vi "SequenceSelector_LoadAllChambers.vi"(5 "Inflow Channel Selector":dbl, 9 "Loop Iteration":i32) -> (4 "Array":u8[][](array[numeric])=[[0, 0, 0, 0, 0, 0, 0, 0, 2, 4, 3, 3, 3, 3], [0, 0, 0, 0, 0, 0, 0, 0, 0, 0, 0, 0, 0, 0], [0, 0, 0, 0, 0, 0, 0, 0, 0, 0, 0, 0, 0, 0], [0, 0, 0, 0, 0, 0, 0, 0, 0, 0, 0, 0, 0, 0], [0, 0, 0, 0, 0, 0, 0, 0, 0, 0, 0, 0, 0, 0], [11, 11, 11, 11, 11, 11, 11, 0, 0, 0, 0, 0, 0, 0], [0, 0, 0, 0, 0, 0, 0, 0, 0, 0, 0, 0, 0, 0], [16, 16, 16, 16, 16, 16, 16, 0, 0, 0, 0, 0, 0, 0], [0, 0, 0, 0, 0, 0, 0, 0, 0, 0, 0, 0, 0, 0], [0, 0, 0, 0, 0, 0, 0, 0, 0, 0, 0, 0, 0, 0], [0, 0, 0, 0, 0, 0, 0, 0, 0, 0, 0, 0, 0, 0], [2, 2, 2, 2, 2, 2, 2, 0, 0, 0, 0, 0, 0, 0], [4, 4, 4, 4, 4, 4, 4, 0, 0, 0, 0, 0, 0, 0], [255, 255, 255, 255, 255, 255, 0, 0, 0, 0, 0, 0, 0, 0], [3, 2, 6, 4, 5, 1, 0, 0, 0, 0, 0, 0, 0, 0], [31, 31, 31, 31, 31, 31, 0, 0, 0, 0, 0, 0, 0, 0], [255, 255, 255, 255, 255, 255, 0, 0, 0, 0, 0, 0, 0, 0]])   [LabVIEW 2016]
panel:
  in  "Byte 4":dbl[](array[numeric])
  in  "Byte 3":dbl[](array[numeric])
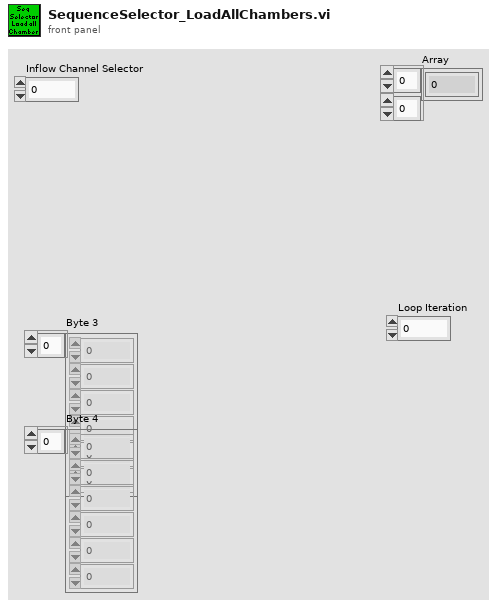
[diagram p1: front panel]
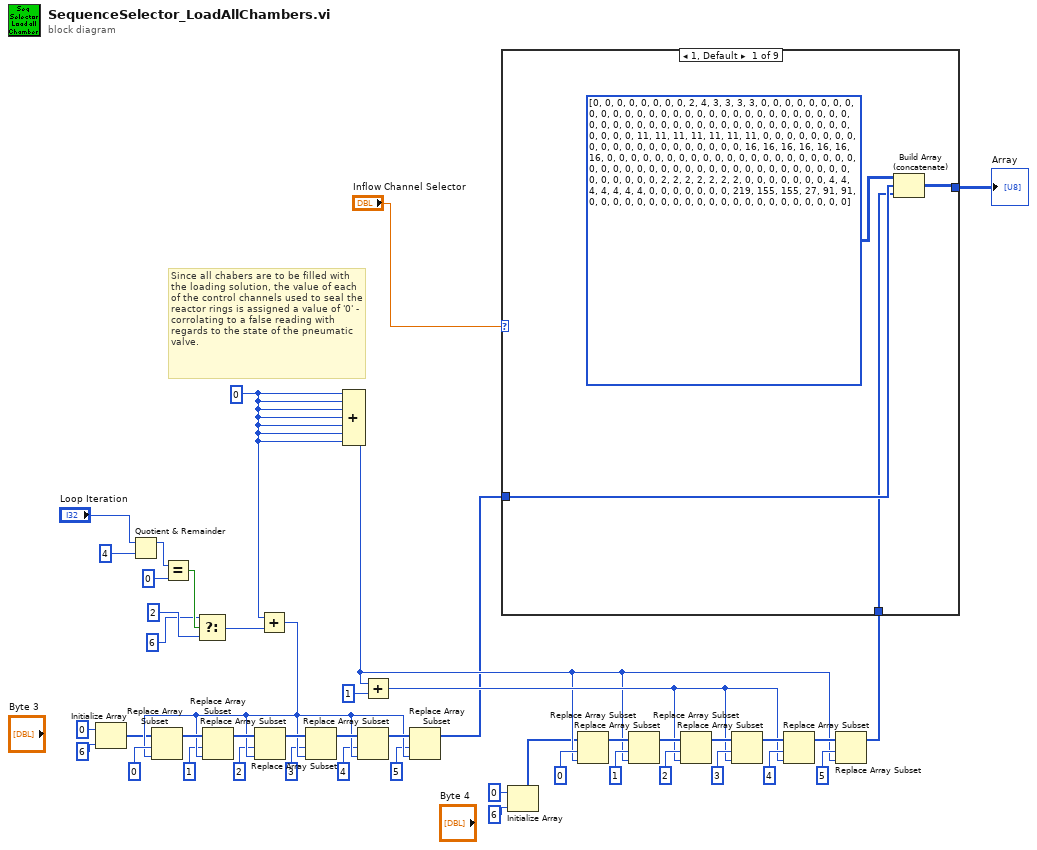
[diagram p0: block diagram]
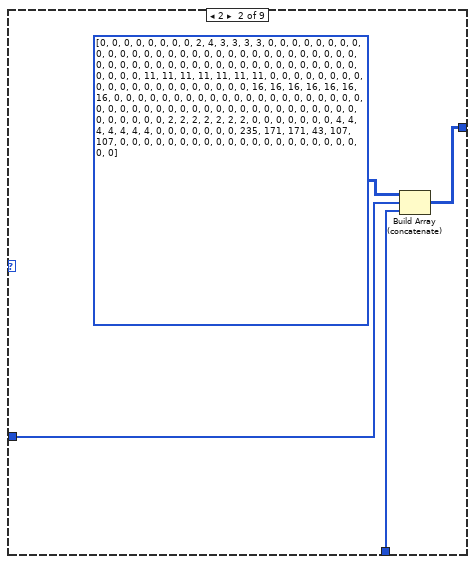
[diagram p2: hidden frame]
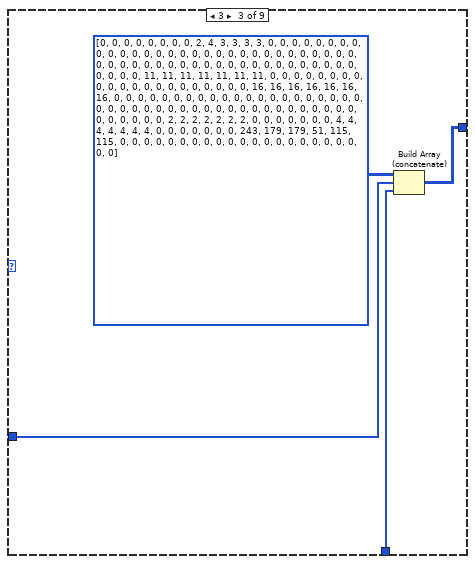
[diagram p3: hidden frame]
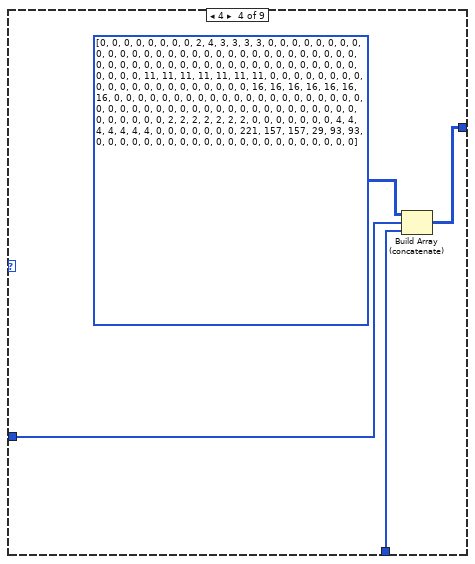
[diagram p4: hidden frame]
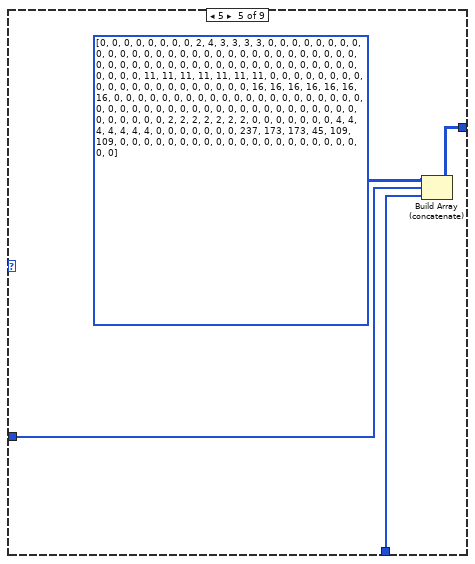
[diagram p5: hidden frame]
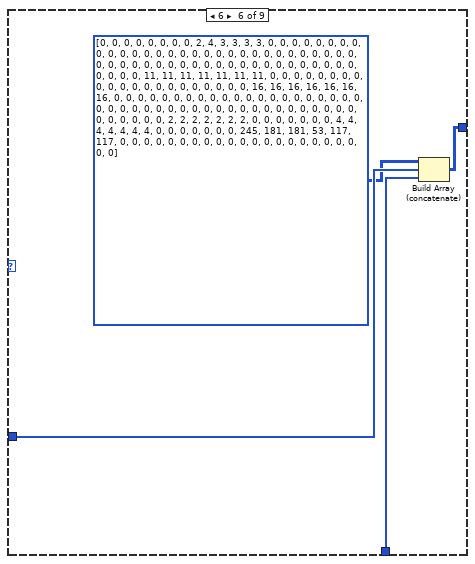
[diagram p6: hidden frame]
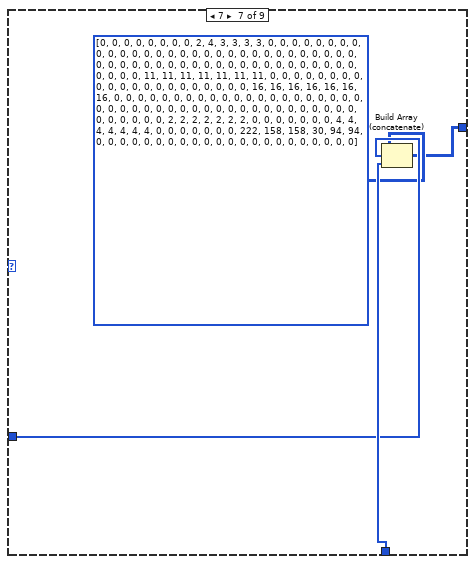
[diagram p7: hidden frame]
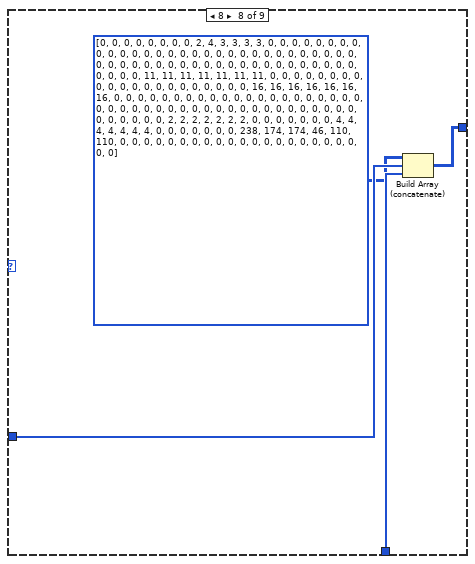
[diagram p8: hidden frame]
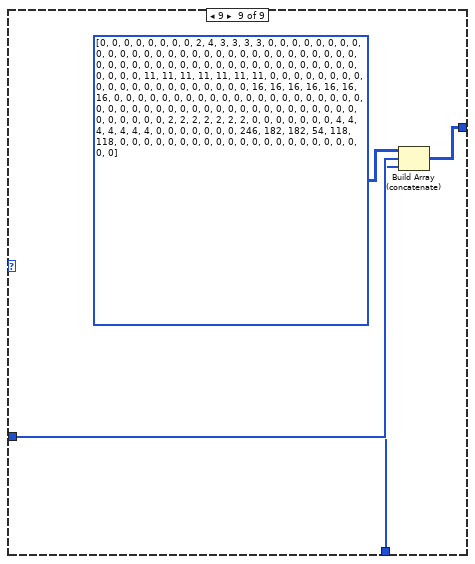
[diagram p9: hidden frame]
diagram:
  w9 = 0
  # "Since all chabers are to be filled with the loading solution, the value of each of the control channels used to seal the reactor rings is assigned a value of '0' - corrolating to a false reading with regards to the state of the pneumatic valve."
  n1 = Initialize Array(0, 6) -> (w10:i32[])
  n2 = Quotient & Remainder(x="Loop Iteration", y=4) -> (x-y*floor(x/y)=w1:i32)  [unwired: 1 out]
  n3 = Equal?(x=w1, y=0) -> (x = y?=w8:bool)
  n4 = Select(t=6, s=w8, f=2) -> (s? t:f=w3:i32)
  n5 = Add(x=w9, y=w3) -> (x+y=w38:i32)
  n6 = Replace Array Subset(array=w10, new element=w38, index=0) -> (w43:i32[])
  n7 = Replace Array Subset(array=w43, new element=w38, index=1) -> (w42:i32[])
  n8 = Replace Array Subset(array=w42, new element=w38, index=2) -> (w41:i32[])
  n9 = Replace Array Subset(array=w41, new element=w38, index=3) -> (w40:i32[])
  n10 = Compound Arithmetic op=unknown(w9, w9, w9, w9, w9, w9, w9) -> (w19:i32)
  n11 = Replace Array Subset(array=w40, new element=w38, index=4) -> (w39:i32[])
  n12 = Add(x=w19, y=1) -> (x+y=w20:i32)
  n13 = Replace Array Subset(array=w39, new element=w38, index=5) -> (w18:i32[])
  n14 = Initialize Array(0, 6) -> (w15:i32[])
  n15 = Replace Array Subset(array=w15, new element=w19, index=0) -> (w23:i32[])
  n16 = Replace Array Subset(array=w23, new element=w19, index=1) -> (w24:i32[])
  n17 = Replace Array Subset(array=w24, new element=w20, index=2) -> (w25:i32[])
  n18 = Replace Array Subset(array=w25, new element=w20, index=3) -> (w26:i32[])
  n19 = Replace Array Subset(array=w26, new element=w20, index=4) -> (w27:i32[])
  n20 = Replace Array Subset(array=w27, new element=w19, index=5) -> (w17:i32[])
  n21 = case shown="1, Default" "Inflow Channel Selector" {
    tunnel: [w49 w50 w54 w58 w65 w69 w70 w74 w80] -> w16
    tunnel: w18 -> [w47 w52 w56 w60 w63 w67 w72 w76 w79]
    tunnel: w17 -> [w46 w53 w57 w61 w64 w68 w73 w77 w78]
    frame 1, Default {
      n22 = Build Array (concatenate)(u8[][] [[0, 0, 0, 0, 0, 0, 0, 0, 2, 4, 3, 3, 3, 3], [0, 0, 0, 0, 0, 0, 0, 0, 0, 0, 0, 0, 0, 0], [0, 0, 0, 0, 0, 0, 0, 0, 0, 0, 0, 0, 0, 0], [0, 0, 0, 0, 0, 0, 0, 0, 0, 0, 0, 0, 0, 0], [0, 0, 0, 0, 0, 0, 0, 0, 0, 0, 0, 0, 0, 0], [11, 11, 11, 11, 11, 11, 11, 0, 0, 0, 0, 0, 0, 0], [0, 0, 0, 0, 0, 0, 0, 0, 0, 0, 0, 0, 0, 0], [16, 16, 16, 16, 16, 16, 16, 0, 0, 0, 0, 0, 0, 0], [0, 0, 0, 0, 0, 0, 0, 0, 0, 0, 0, 0, 0, 0], [0, 0, 0, 0, 0, 0, 0, 0, 0, 0, 0, 0, 0, 0], [0, 0, 0, 0, 0, 0, 0, 0, 0, 0, 0, 0, 0, 0], [2, 2, 2, 2, 2, 2, 2, 0, 0, 0, 0, 0, 0, 0], [4, 4, 4, 4, 4, 4, 4, 0, 0, 0, 0, 0, 0, 0], [219, 155, 155, 27, 91, 91, 0, 0, 0, 0, 0, 0, 0, 0], [0, 0, 0, 0, 0, 0, 0, 0, 0, 0, 0, 0, 0, 0]], w47, w46) -> (w49:i32[][])
    }
    frame 2 {
      n23 = Build Array (concatenate)(u8[][] [[0, 0, 0, 0, 0, 0, 0, 0, 2, 4, 3, 3, 3, 3], [0, 0, 0, 0, 0, 0, 0, 0, 0, 0, 0, 0, 0, 0], [0, 0, 0, 0, 0, 0, 0, 0, 0, 0, 0, 0, 0, 0], [0, 0, 0, 0, 0, 0, 0, 0, 0, 0, 0, 0, 0, 0], [0, 0, 0, 0, 0, 0, 0, 0, 0, 0, 0, 0, 0, 0], [11, 11, 11, 11, 11, 11, 11, 0, 0, 0, 0, 0, 0, 0], [0, 0, 0, 0, 0, 0, 0, 0, 0, 0, 0, 0, 0, 0], [16, 16, 16, 16, 16, 16, 16, 0, 0, 0, 0, 0, 0, 0], [0, 0, 0, 0, 0, 0, 0, 0, 0, 0, 0, 0, 0, 0], [0, 0, 0, 0, 0, 0, 0, 0, 0, 0, 0, 0, 0, 0], [0, 0, 0, 0, 0, 0, 0, 0, 0, 0, 0, 0, 0, 0], [2, 2, 2, 2, 2, 2, 2, 0, 0, 0, 0, 0, 0, 0], [4, 4, 4, 4, 4, 4, 4, 0, 0, 0, 0, 0, 0, 0], [235, 171, 171, 43, 107, 107, 0, 0, 0, 0, 0, 0, 0, 0], [0, 0, 0, 0, 0, 0, 0, 0, 0, 0, 0, 0, 0, 0]], w52, w53) -> (w50:i32[][])
    }
    frame 3 {
      n24 = Build Array (concatenate)(u8[][] [[0, 0, 0, 0, 0, 0, 0, 0, 2, 4, 3, 3, 3, 3], [0, 0, 0, 0, 0, 0, 0, 0, 0, 0, 0, 0, 0, 0], [0, 0, 0, 0, 0, 0, 0, 0, 0, 0, 0, 0, 0, 0], [0, 0, 0, 0, 0, 0, 0, 0, 0, 0, 0, 0, 0, 0], [0, 0, 0, 0, 0, 0, 0, 0, 0, 0, 0, 0, 0, 0], [11, 11, 11, 11, 11, 11, 11, 0, 0, 0, 0, 0, 0, 0], [0, 0, 0, 0, 0, 0, 0, 0, 0, 0, 0, 0, 0, 0], [16, 16, 16, 16, 16, 16, 16, 0, 0, 0, 0, 0, 0, 0], [0, 0, 0, 0, 0, 0, 0, 0, 0, 0, 0, 0, 0, 0], [0, 0, 0, 0, 0, 0, 0, 0, 0, 0, 0, 0, 0, 0], [0, 0, 0, 0, 0, 0, 0, 0, 0, 0, 0, 0, 0, 0], [2, 2, 2, 2, 2, 2, 2, 0, 0, 0, 0, 0, 0, 0], [4, 4, 4, 4, 4, 4, 4, 0, 0, 0, 0, 0, 0, 0], [243, 179, 179, 51, 115, 115, 0, 0, 0, 0, 0, 0, 0, 0], [0, 0, 0, 0, 0, 0, 0, 0, 0, 0, 0, 0, 0, 0]], w56, w57) -> (w54:i32[][])
    }
    frame 4 {
      n25 = Build Array (concatenate)(u8[][] [[0, 0, 0, 0, 0, 0, 0, 0, 2, 4, 3, 3, 3, 3], [0, 0, 0, 0, 0, 0, 0, 0, 0, 0, 0, 0, 0, 0], [0, 0, 0, 0, 0, 0, 0, 0, 0, 0, 0, 0, 0, 0], [0, 0, 0, 0, 0, 0, 0, 0, 0, 0, 0, 0, 0, 0], [0, 0, 0, 0, 0, 0, 0, 0, 0, 0, 0, 0, 0, 0], [11, 11, 11, 11, 11, 11, 11, 0, 0, 0, 0, 0, 0, 0], [0, 0, 0, 0, 0, 0, 0, 0, 0, 0, 0, 0, 0, 0], [16, 16, 16, 16, 16, 16, 16, 0, 0, 0, 0, 0, 0, 0], [0, 0, 0, 0, 0, 0, 0, 0, 0, 0, 0, 0, 0, 0], [0, 0, 0, 0, 0, 0, 0, 0, 0, 0, 0, 0, 0, 0], [0, 0, 0, 0, 0, 0, 0, 0, 0, 0, 0, 0, 0, 0], [2, 2, 2, 2, 2, 2, 2, 0, 0, 0, 0, 0, 0, 0], [4, 4, 4, 4, 4, 4, 4, 0, 0, 0, 0, 0, 0, 0], [221, 157, 157, 29, 93, 93, 0, 0, 0, 0, 0, 0, 0, 0], [0, 0, 0, 0, 0, 0, 0, 0, 0, 0, 0, 0, 0, 0]], w60, w61) -> (w58:i32[][])
    }
    frame 5 {
      n26 = Build Array (concatenate)(u8[][] [[0, 0, 0, 0, 0, 0, 0, 0, 2, 4, 3, 3, 3, 3], [0, 0, 0, 0, 0, 0, 0, 0, 0, 0, 0, 0, 0, 0], [0, 0, 0, 0, 0, 0, 0, 0, 0, 0, 0, 0, 0, 0], [0, 0, 0, 0, 0, 0, 0, 0, 0, 0, 0, 0, 0, 0], [0, 0, 0, 0, 0, 0, 0, 0, 0, 0, 0, 0, 0, 0], [11, 11, 11, 11, 11, 11, 11, 0, 0, 0, 0, 0, 0, 0], [0, 0, 0, 0, 0, 0, 0, 0, 0, 0, 0, 0, 0, 0], [16, 16, 16, 16, 16, 16, 16, 0, 0, 0, 0, 0, 0, 0], [0, 0, 0, 0, 0, 0, 0, 0, 0, 0, 0, 0, 0, 0], [0, 0, 0, 0, 0, 0, 0, 0, 0, 0, 0, 0, 0, 0], [0, 0, 0, 0, 0, 0, 0, 0, 0, 0, 0, 0, 0, 0], [2, 2, 2, 2, 2, 2, 2, 0, 0, 0, 0, 0, 0, 0], [4, 4, 4, 4, 4, 4, 4, 0, 0, 0, 0, 0, 0, 0], [237, 173, 173, 45, 109, 109, 0, 0, 0, 0, 0, 0, 0, 0], [0, 0, 0, 0, 0, 0, 0, 0, 0, 0, 0, 0, 0, 0]], w63, w64) -> (w65:i32[][])
    }
    frame 6 {
      n27 = Build Array (concatenate)(u8[][] [[0, 0, 0, 0, 0, 0, 0, 0, 2, 4, 3, 3, 3, 3], [0, 0, 0, 0, 0, 0, 0, 0, 0, 0, 0, 0, 0, 0], [0, 0, 0, 0, 0, 0, 0, 0, 0, 0, 0, 0, 0, 0], [0, 0, 0, 0, 0, 0, 0, 0, 0, 0, 0, 0, 0, 0], [0, 0, 0, 0, 0, 0, 0, 0, 0, 0, 0, 0, 0, 0], [11, 11, 11, 11, 11, 11, 11, 0, 0, 0, 0, 0, 0, 0], [0, 0, 0, 0, 0, 0, 0, 0, 0, 0, 0, 0, 0, 0], [16, 16, 16, 16, 16, 16, 16, 0, 0, 0, 0, 0, 0, 0], [0, 0, 0, 0, 0, 0, 0, 0, 0, 0, 0, 0, 0, 0], [0, 0, 0, 0, 0, 0, 0, 0, 0, 0, 0, 0, 0, 0], [0, 0, 0, 0, 0, 0, 0, 0, 0, 0, 0, 0, 0, 0], [2, 2, 2, 2, 2, 2, 2, 0, 0, 0, 0, 0, 0, 0], [4, 4, 4, 4, 4, 4, 4, 0, 0, 0, 0, 0, 0, 0], [245, 181, 181, 53, 117, 117, 0, 0, 0, 0, 0, 0, 0, 0], [0, 0, 0, 0, 0, 0, 0, 0, 0, 0, 0, 0, 0, 0]], w67, w68) -> (w69:i32[][])
    }
    frame 7 {
      n28 = Build Array (concatenate)(u8[][] [[0, 0, 0, 0, 0, 0, 0, 0, 2, 4, 3, 3, 3, 3], [0, 0, 0, 0, 0, 0, 0, 0, 0, 0, 0, 0, 0, 0], [0, 0, 0, 0, 0, 0, 0, 0, 0, 0, 0, 0, 0, 0], [0, 0, 0, 0, 0, 0, 0, 0, 0, 0, 0, 0, 0, 0], [0, 0, 0, 0, 0, 0, 0, 0, 0, 0, 0, 0, 0, 0], [11, 11, 11, 11, 11, 11, 11, 0, 0, 0, 0, 0, 0, 0], [0, 0, 0, 0, 0, 0, 0, 0, 0, 0, 0, 0, 0, 0], [16, 16, 16, 16, 16, 16, 16, 0, 0, 0, 0, 0, 0, 0], [0, 0, 0, 0, 0, 0, 0, 0, 0, 0, 0, 0, 0, 0], [0, 0, 0, 0, 0, 0, 0, 0, 0, 0, 0, 0, 0, 0], [0, 0, 0, 0, 0, 0, 0, 0, 0, 0, 0, 0, 0, 0], [2, 2, 2, 2, 2, 2, 2, 0, 0, 0, 0, 0, 0, 0], [4, 4, 4, 4, 4, 4, 4, 0, 0, 0, 0, 0, 0, 0], [222, 158, 158, 30, 94, 94, 0, 0, 0, 0, 0, 0, 0, 0], [0, 0, 0, 0, 0, 0, 0, 0, 0, 0, 0, 0, 0, 0]], w72, w73) -> (w70:i32[][])
    }
    frame 8 {
      n29 = Build Array (concatenate)(u8[][] [[0, 0, 0, 0, 0, 0, 0, 0, 2, 4, 3, 3, 3, 3], [0, 0, 0, 0, 0, 0, 0, 0, 0, 0, 0, 0, 0, 0], [0, 0, 0, 0, 0, 0, 0, 0, 0, 0, 0, 0, 0, 0], [0, 0, 0, 0, 0, 0, 0, 0, 0, 0, 0, 0, 0, 0], [0, 0, 0, 0, 0, 0, 0, 0, 0, 0, 0, 0, 0, 0], [11, 11, 11, 11, 11, 11, 11, 0, 0, 0, 0, 0, 0, 0], [0, 0, 0, 0, 0, 0, 0, 0, 0, 0, 0, 0, 0, 0], [16, 16, 16, 16, 16, 16, 16, 0, 0, 0, 0, 0, 0, 0], [0, 0, 0, 0, 0, 0, 0, 0, 0, 0, 0, 0, 0, 0], [0, 0, 0, 0, 0, 0, 0, 0, 0, 0, 0, 0, 0, 0], [0, 0, 0, 0, 0, 0, 0, 0, 0, 0, 0, 0, 0, 0], [2, 2, 2, 2, 2, 2, 2, 0, 0, 0, 0, 0, 0, 0], [4, 4, 4, 4, 4, 4, 4, 0, 0, 0, 0, 0, 0, 0], [238, 174, 174, 46, 110, 110, 0, 0, 0, 0, 0, 0, 0, 0], [0, 0, 0, 0, 0, 0, 0, 0, 0, 0, 0, 0, 0, 0]], w76, w77) -> (w74:i32[][])
    }
    frame 9 {
      n30 = Build Array (concatenate)(u8[][] [[0, 0, 0, 0, 0, 0, 0, 0, 2, 4, 3, 3, 3, 3], [0, 0, 0, 0, 0, 0, 0, 0, 0, 0, 0, 0, 0, 0], [0, 0, 0, 0, 0, 0, 0, 0, 0, 0, 0, 0, 0, 0], [0, 0, 0, 0, 0, 0, 0, 0, 0, 0, 0, 0, 0, 0], [0, 0, 0, 0, 0, 0, 0, 0, 0, 0, 0, 0, 0, 0], [11, 11, 11, 11, 11, 11, 11, 0, 0, 0, 0, 0, 0, 0], [0, 0, 0, 0, 0, 0, 0, 0, 0, 0, 0, 0, 0, 0], [16, 16, 16, 16, 16, 16, 16, 0, 0, 0, 0, 0, 0, 0], [0, 0, 0, 0, 0, 0, 0, 0, 0, 0, 0, 0, 0, 0], [0, 0, 0, 0, 0, 0, 0, 0, 0, 0, 0, 0, 0, 0], [0, 0, 0, 0, 0, 0, 0, 0, 0, 0, 0, 0, 0, 0], [2, 2, 2, 2, 2, 2, 2, 0, 0, 0, 0, 0, 0, 0], [4, 4, 4, 4, 4, 4, 4, 0, 0, 0, 0, 0, 0, 0], [246, 182, 182, 54, 118, 118, 0, 0, 0, 0, 0, 0, 0, 0], [0, 0, 0, 0, 0, 0, 0, 0, 0, 0, 0, 0, 0, 0]], w79, w78) -> (w80:i32[][])
    }
  }
  "Array" <- w16
